vi "Feeder State Machine.vi"(6 "elapsed time(s)":dbl, 9 "state data in":T3={"timer"=0.0, "hopper level"=10, "servings to dispense"=0, "clock time"=21601.0, "last dispense time"=0.0, "program mode"="none", "schedule"=[{"time"="6:00 am", "servings"=2}, {"time"="7:00 am", "servings"=3}, {"time"="11:00 am", "servings"=4}, {"time"="12:00 am", "servings"=99}]} {"last dispense time" format="%<%H:%M:%S>t"; "clock time" format="%<%H:%M:%S>t"}, 10 "state machine event":T2, 11 "state in":T1) -> (1 "state data out":T3 {"last dispense time" format="%<%H:%M:%S>t"; "clock time" format="%<%H:%M:%S>t"}, 3 "state out":T1)   [LabVIEW 2019, in "Pet Feeder.lvlib"]
doc: "This SubVI contains the primary logic for the automated pet feeder. \n\nThis VI should not have any side-effects on the appliction (it performs no I/O). This means that this VI can be easily unit tested."
uses:
  Pet Feeder.lvlib
  Types/internal_state_data.ctl
  Controls/Feeder Program.ctl
  Types/state_machine_event.ctl
  Types/state.ctl
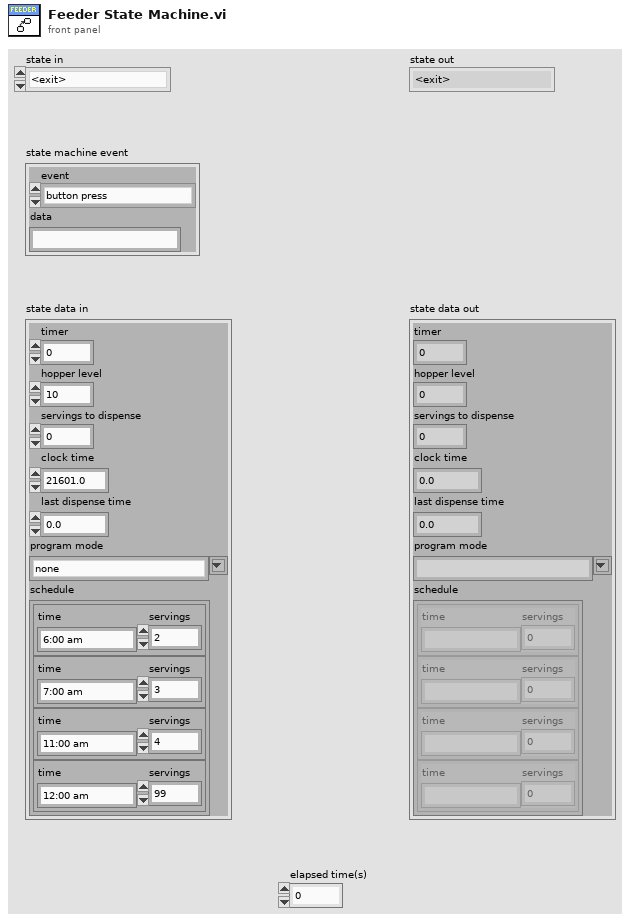
[diagram p1: front panel]
types:
  T1 = typedef "Pet Feeder.lvlib/state.ctl" = enum16{"<exit>", "<entry>", "idle", "dispensing"}
  T2 = typedef "Pet Feeder.lvlib/state_machine_event.ctl" = cluster{"event":enum16{"button press", "timeout"}, "data":string}
  T3 = typedef "Pet Feeder.lvlib/internal_state_data.ctl" = cluster{"timer":dbl, "hopper level":i32, "servings to dispense":i32, "clock time":dbl, "last dispense time":dbl, "program mode":string, "schedule":T4[]}
  T4 = typedef "Pet Feeder.lvlib/Feeder Program.ctl" = cluster{"time":string, "servings":i32}
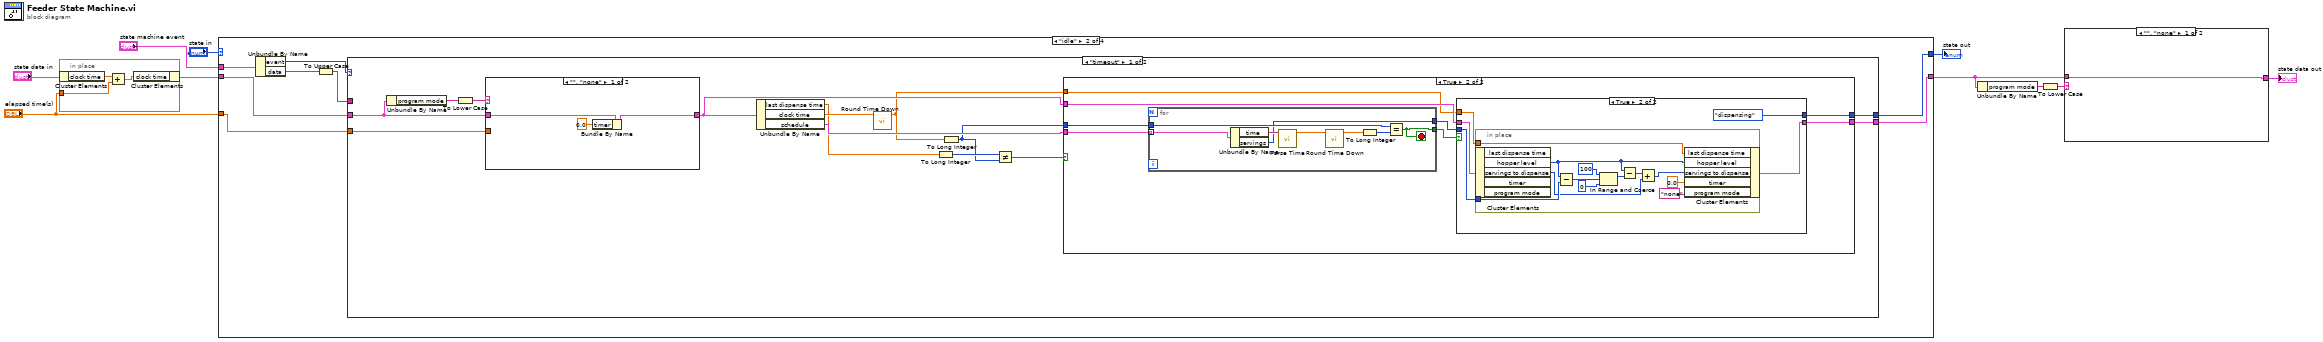
[diagram p0: block diagram]
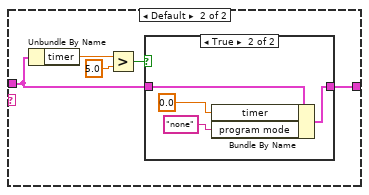
[diagram p2: hidden frame]
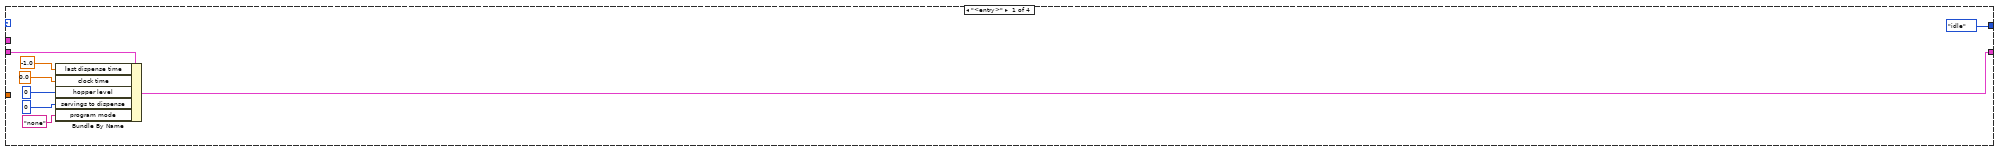
[diagram p4: hidden frame]
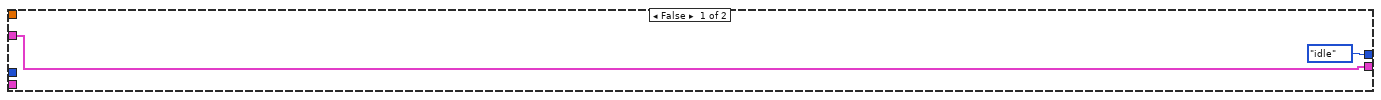
[diagram p5: hidden frame]
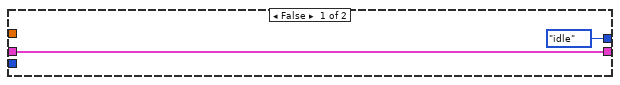
[diagram p6: hidden frame]
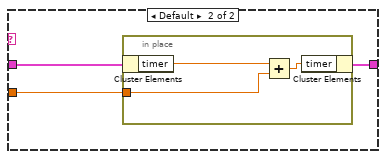
[diagram p7: hidden frame]
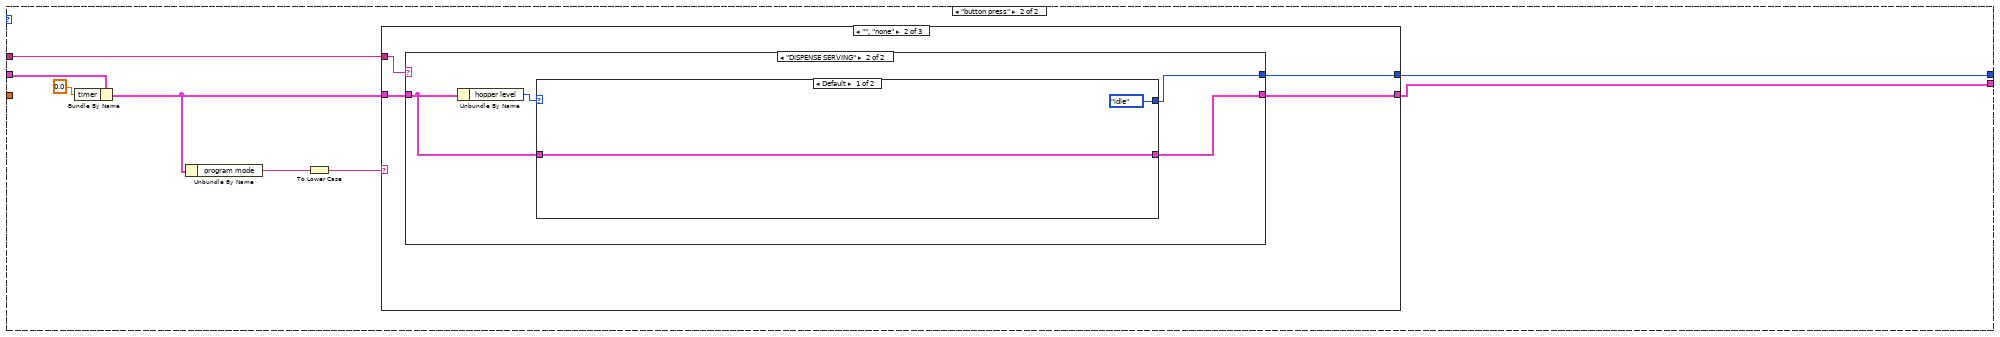
[diagram p8: hidden frame]
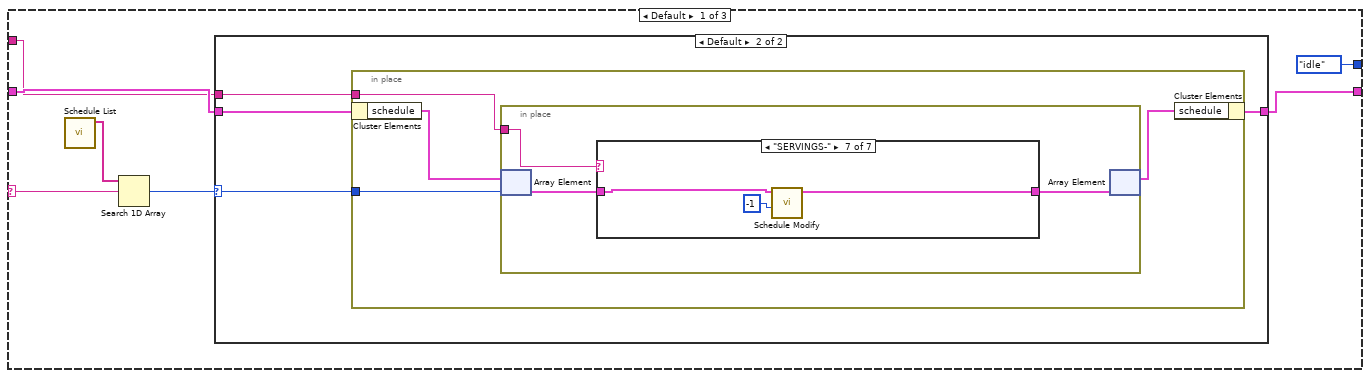
[diagram p9: hidden frame]
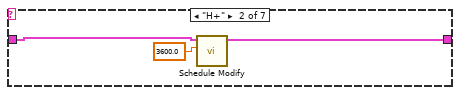
[diagram p12: hidden frame]
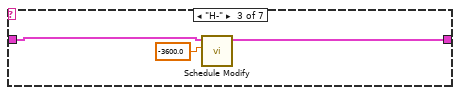
[diagram p13: hidden frame]
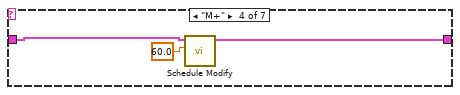
[diagram p14: hidden frame]
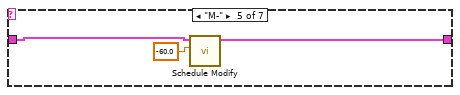
[diagram p15: hidden frame]
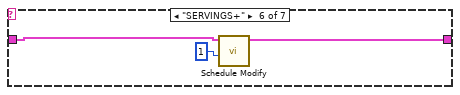
[diagram p16: hidden frame]
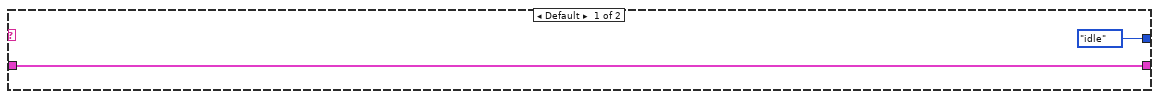
[diagram p17: hidden frame]
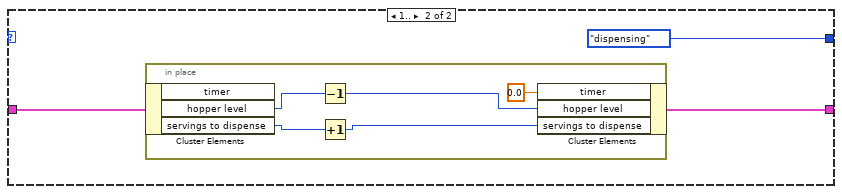
[diagram p18: hidden frame]
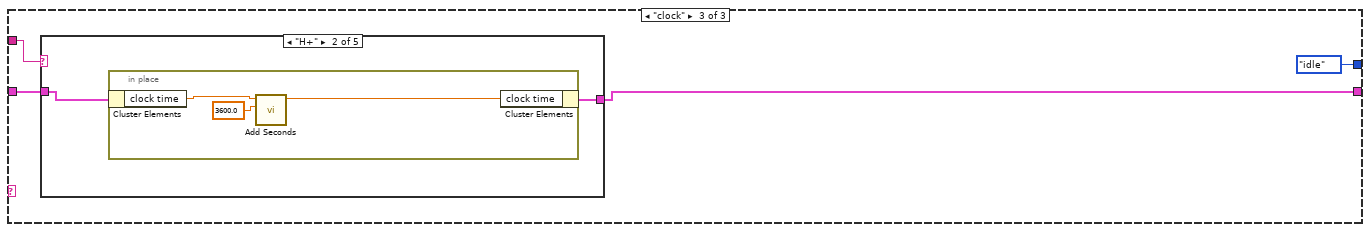
[diagram p19: hidden frame]
diagram:
  n1 = in-place {
    in-place-border: "elapsed time(s)" -> [w12]
    n2 = in-place-cluster #1("state data in") -> ("clock time"=w13:dbl)
    n3 = Add(x=w13, y=w12) -> (x+y=w11:dbl)
    n4 = in-place-cluster #1("clock time"=w11) -> (w6:T3)
  }
  n5 = case shown="\"idle\"" "state in" {
    tunnel: [state."idle" ("state in") w22 w186 state."<exit>" ("state in")] -> w8
    tunnel: "state machine event" -> [_ w29 _ _]
    tunnel: [w19 w24 w184 w212] -> w2
    tunnel: w6 -> [w20 w26 w196 w212]
    tunnel: "elapsed time(s)" -> [_ w23 w195 _]
    frame "<entry>" {
      n6 = Bundle By Name(cluster=w20, "last dispense time"=-1.0, "clock time"=0.0, "hopper level"=0, "servings to dispense"=0, "program mode"="none") -> (w19:T3)
    }
    frame "idle" {
      n7 = Unbundle By Name(w29) -> ("event"=w28:enum16{"button press", "timeout"}, "data"=w27:string)
      n8 = To Upper Case(1:w27) -> (0:w25:string)
      n9 = case shown="\"timeout\"" w28 {
        tunnel: w25 -> [_ w97]
        tunnel: w26 -> [w41 w94]
        tunnel: [w33 w93] -> w24
        tunnel: w23 -> [w40 _]
        tunnel: [w31 w90] -> w22
        frame "timeout" {
          n10 = Unbundle By Name(w41) -> ("program mode"=w43:string)
          n11 = To Lower Case(string=w43) -> (all lower case string=w42:string)
          n12 = case shown="\"\", \"none\"" w42 {
            tunnel: w41 -> [w83 w86]
            tunnel: w40 -> [_ w85]
            tunnel: [w82 w84] -> w34
            frame "", "none" {
              n13 = Bundle By Name(cluster=w83, "timer"=0.0) -> (w82:T3)
            }
            frame Default {
              n14 = in-place {
                in-place-border: w85 -> [w87]
                n15 = in-place-cluster #2(w86) -> ("timer"=w89:dbl)
                n16 = Add(x=w89, y=w87) -> (x+y=w88:dbl)
                n17 = in-place-cluster #2("timer"=w88) -> (w84:T3)
              }
            }
          }
          n18 = Unbundle By Name(w34) -> ("last dispense time"=w37:dbl, "clock time"=w38:dbl, "schedule"=w39:T4[])
          n19 = call "Round Time Down.vi"("clock time"=w38) -> ("lower minute"=w30:dbl)  [unwired: 10 in]
          n20 = To Long Integer(number=w37) -> (32bit integer=w36:i32)
          n21 = To Long Integer(number=w30) -> (32bit integer=w32:i32)
          n22 = Not Equal?(x=w36, y=w32) -> (x != y?=w35:bool)
          n23 = case shown="True" w35 {
            tunnel: w39 -> [_ w53]
            tunnel: [w45 w50] -> w33
            tunnel: w34 -> [w45 w49]
            tunnel: w32 -> [_ w52]
            tunnel: [state."idle" ("state in") w47] -> w31
            tunnel: w30 -> [_ w46]
            frame False {
            }
            frame True {
              n24 = for {
                tunnel: w53 -> [w80] mode=indexing
                tunnel: w52 -> [w75]
                tunnel: [w74] -> w48
                tunnel: [w73] -> w51
                stop <- w73 stop-if-true
                n25 = Unbundle By Name(w80) -> ("time"=w79:string, "servings"=w74:i32)
                n26 = call "Parse Time.vi"("parse time"=w79) -> ("time (HH:MM:SS)"=w78:dbl)  [unwired: 10 in]
                n27 = call "Round Time Down.vi"("clock time"=w78) -> ("lower minute"=w77:dbl)  [unwired: 10 in]
                n28 = To Long Integer(number=w77) -> (32bit integer=w76:i32)
                n29 = Equal?(x=w75, y=w76) -> (x = y?=w73:bool)
              }
              n30 = case shown="True" w51 {
                tunnel: [w55 w58] -> w50
                tunnel: w49 -> [w55 w60]
                tunnel: w48 -> [_ w59]
                tunnel: [state."idle" ("state in") state."dispensing" ("state in")] -> w47
                tunnel: w46 -> [_ w56]
                frame False {
                }
                frame True {
                  n31 = in-place {
                    in-place-border: w59 -> [w72]
                    in-place-border: w56 -> [w63]
                    n32 = in-place-cluster #3(w60) -> ("hopper level"=w62:i32, "servings to dispense"=w65:i32)  [unwired: 3 out]
                    n33 = Subtract(x=w62, y=w72) -> (x-y=w71:i32)
                    n34 = In Range and Coerce(upper limit=100, x=w71, lower limit=0 ("upper limit")) -> (coerced(x)=w68:i32)  [unwired: 1 out]
                    n35 = Subtract(x=w62, y=w68) -> (x-y=w67:i32)
                    n36 = Add(x=w67, y=w65) -> (x+y=w66:i32)
                    n37 = in-place-cluster #3("last dispense time"=w63, "hopper level"=w62, "servings to dispense"=w66, "timer"=0.0, "program mode"="none") -> (w58:T3)
                  }
                }
              }
            }
          }
        }
        frame "button press" {
          n38 = Bundle By Name(cluster=w94, "timer"=0.0) -> (w92:T3)
          n39 = Unbundle By Name(w92) -> ("program mode"=w96:string)
          n40 = To Lower Case(string=w96) -> (all lower case string=w95:string)
          n41 = case shown="\"\", \"none\"" w95 {
            selector: w95 -> [w103 _ _]
            tunnel: w97 -> [w99 w139 w159]
            tunnel: w92 -> [w101 w138 w158]
            tunnel: [w100 w137 w157] -> w93
            tunnel: [state."idle" ("state in") w136 state."idle" ("state in")] -> w90
            frame Default {
              n42 = call "Schedule List.vi"() -> ("schedules"=w104:string[])  [unwired: 11 in]
              n43 = Search 1D Array(1D array=w104, element=w103) -> (index of element=w102:i32)  [unwired: 1 in]
              n44 = case shown="Default" w102 {
                selector: w102 -> [_ w108]
                tunnel: [w105 w106] -> w100
                tunnel: w101 -> [w105 w109]
                tunnel: w99 -> [_ w107]
                frame -1 {
                }
                frame Default {
                  n45 = in-place {
                    in-place-border: w108 -> [w112]
                    in-place-border: w107 -> [w111]
                    n46 = in-place-cluster #4(w109) -> ("schedule"=w113:T4[])
                    n47 = in-place {
                      in-place-border: w111 -> [w116]
                      n48 = in-place-array #5(w113, w112) -> (w115:T4)
                      n49 = case shown="\"SERVINGS-\"" w116 {
                        tunnel: w115 -> [w117 w120 w123 w126 w129 w132 w135]
                        tunnel: [w117 w119 w122 w125 w128 w131 w134] -> w114
                        frame Default {
                        }
                        frame "H+" {
                          n50 = call "Schedule Modify.vi"("seconds"=3600.0 ("y"), "sched in"=w120) -> ("sched out"=w119:T4)  [unwired: 9 in]
                        }
                        frame "H-" {
                          n51 = call "Schedule Modify.vi"("seconds"=-3600.0 ("y"), "sched in"=w123) -> ("sched out"=w122:T4)  [unwired: 9 in]
                        }
                        frame "M+" {
                          n52 = call "Schedule Modify.vi"("seconds"=60.0 ("y"), "sched in"=w126) -> ("sched out"=w125:T4)  [unwired: 9 in]
                        }
                        frame "M-" {
                          n53 = call "Schedule Modify.vi"("seconds"=-60.0 ("y"), "sched in"=w129) -> ("sched out"=w128:T4)  [unwired: 9 in]
                        }
                        frame "SERVINGS+" {
                          n54 = call "Schedule Modify.vi"("servings"=1, "sched in"=w132) -> ("sched out"=w131:T4)  [unwired: 9 in]
                        }
                        frame "SERVINGS-" {
                          n55 = call "Schedule Modify.vi"("servings"=-1, "sched in"=w135) -> ("sched out"=w134:T4)  [unwired: 9 in]
                        }
                      }
                      n56 = in-place-array #5(w114) -> (w110:T4[])  [unwired: 1 out]
                    }
                    n57 = in-place-cluster #4("schedule"=w110) -> (w106:T3)
                  }
                }
              }
            }
            frame "", "none" {
              n58 = case shown="\"DISPENSE SERVING\"" w139 {
                tunnel: w138 -> [w141 w145]
                tunnel: [w141 w143] -> w137
                tunnel: [state."idle" ("state in") w142] -> w136
                frame Default {
                }
                frame "DISPENSE SERVING" {
                  n59 = Unbundle By Name(w145) -> ("hopper level"=w144:i32)
                  n60 = case shown="Default" w144 {
                    tunnel: w145 -> [w147 w150]
                    tunnel: [w147 w149] -> w143
                    tunnel: [state."idle" ("state in") state."dispensing" ("state in")] -> w142
                    frame Default {
                    }
                    frame 1.. {
                      n61 = in-place {
                        n62 = in-place-cluster #6(w150) -> ("hopper level"=w154:i32, "servings to dispense"=w152:i32)  [unwired: 1 out]
                        n63 = Decrement(x=w154) -> (x-1=w153:i32)
                        n64 = Increment(x=w152) -> (x+1=w151:i32)
                        n65 = in-place-cluster #6("timer"=0.0, "hopper level"=w153, "servings to dispense"=w151) -> (w149:T3)
                      }
                    }
                  }
                }
              }
            }
            frame "clock" {
              n66 = case shown="\"H+\"" w159 {
                tunnel: w158 -> [w160 w162 w167 w172 w178]
                tunnel: [w160 w161 w166 w171 w177] -> w157
                frame Default {
                }
                frame "H+" {
                  n67 = in-place {
                    n68 = in-place-cluster #7(w162) -> ("clock time"=w165:dbl)
                    n69 = call "Add Seconds.vi"("seconds"=3600.0 ("y"), "time in"=w165) -> ("time out"=w163:dbl)  [unwired: 9 in]
                    n70 = in-place-cluster #7("clock time"=w163) -> (w161:T3)
                  }
                }
                frame "H-" {
                  n71 = in-place {
                    n72 = in-place-cluster #8(w167) -> ("clock time"=w170:dbl)
                    n73 = call "Add Seconds.vi"("seconds"=-3600.0 ("y"), "time in"=w170) -> ("time out"=w168:dbl)  [unwired: 9 in]
                    n74 = in-place-cluster #8("clock time"=w168) -> (w166:T3)
                  }
                }
                frame "M+" {
                  n75 = in-place {
                    n76 = in-place-cluster #9(w172) -> ("clock time"=w176:dbl)
                    n77 = call "Add Seconds.vi"("reset minute?"=TRUE, "seconds"=60.0 ("y"), "time in"=w176) -> ("time out"=w174:dbl)  [unwired: 8 in]
                    n78 = in-place-cluster #9("clock time"=w174) -> (w171:T3)
                  }
                }
                frame "M-" {
                  n79 = in-place {
                    n80 = in-place-cluster #10(w178) -> ("clock time"=w182:dbl)
                    n81 = call "Add Seconds.vi"("reset minute?"=TRUE, "seconds"=-60.0 ("y"), "time in"=w182) -> ("time out"=w180:dbl)  [unwired: 8 in]
                    n82 = in-place-cluster #10("clock time"=w180) -> (w177:T3)
                  }
                }
              }
            }
          }
        }
      }
    }
    frame "dispensing" {
      n83 = in-place {
        in-place-border: w195 -> [w210]
        n84 = in-place-cluster #11(w196) -> ("timer"=w211:dbl)
        n85 = Add(x=w211, y=w210) -> (x+y=w209:dbl)
        n86 = in-place-cluster #11("timer"=w209) -> (w191:T3)
      }
      n87 = Unbundle By Name(w191) -> ("timer"=w194:dbl)
      n88 = Greater Or Equal?(x=w194, y=5.0) -> (x >= y?=w192:bool)
      n89 = case shown="True" w192 {
        tunnel: w191 -> [w197 w199]
        tunnel: [w197 w198] -> w185
        frame False {
        }
        frame True {
          n90 = in-place {
            n91 = in-place-cluster #12(w199) -> ("servings to dispense"=w204:i32, "hopper level"=w202:i32)  [unwired: 1 out]
            n92 = Decrement(x=w204) -> (x-1=w208:i32)
            n93 = In Range and Coerce(upper limit=100, x=w208, lower limit=0 ("x-1")) -> (coerced(x)=w203:i32)  [unwired: 1 out]
            n94 = Subtract(x=w204, y=w203) -> (x-y=w201:i32)
            n95 = Subtract(x=w202, y=w201) -> (x-y=w200:i32)
            n96 = in-place-cluster #12("timer"=0.0, "servings to dispense"=w203, "hopper level"=w200) -> (w198:T3)
          }
        }
      }
      n97 = Unbundle By Name(w185) -> ("servings to dispense"=w190:i32)
      n98 = Greater Than 0?(x=w190) -> (x > 0?=w189:bool)
      n99 = Select(t=state."dispensing" ("state in"), s=w189, f=state."idle" ("state in")) -> (s? t:f=w186:T1)
      n100 = Bundle By Name(cluster=w185, "program mode"="none") -> (w184:T3)
    }
    frame "<exit>" {
    }
  }
  "state out" <- w8
  n101 = Unbundle By Name(w2) -> ("program mode"=w4:string)
  n102 = To Lower Case(string=w4) -> (all lower case string=w3:string)
  n103 = case shown="\"\", \"none\"" w3 {
    tunnel: [w214 w215] -> w1
    tunnel: w2 -> [w214 w216]
    frame "", "none" {
    }
    frame Default {
      n104 = Unbundle By Name(w216) -> ("timer"=w219:dbl)
      n105 = Greater?(x=w219, y=5.0) -> (0:w217:bool)
      n106 = case shown="True" w217 {
        tunnel: w216 -> [w220 w224]
        tunnel: [w220 w221] -> w215
        frame False {
        }
        frame True {
          n107 = Bundle By Name(cluster=w224, "timer"=0.0, "program mode"="none") -> (w221:T3)
        }
      }
    }
  }
  "state data out" <- w1
